vi "User Message Event Callback.vi"(4 "TS UI Data":T1, 5 "Event Data":cluster{"uiMsg":refnum<k7>}, 6 "Control Ref":refnum<k7>, 7 "Event Common Data":T2) -> ()   [LabVIEW 2015]
uses:
  Type defs/TS UI Data.ctl
  Type defs/Nest cluster.ctl
panel:
  # "SCANNED DATA"
  # "ITAC DATA"
  # "DoIP DATA"
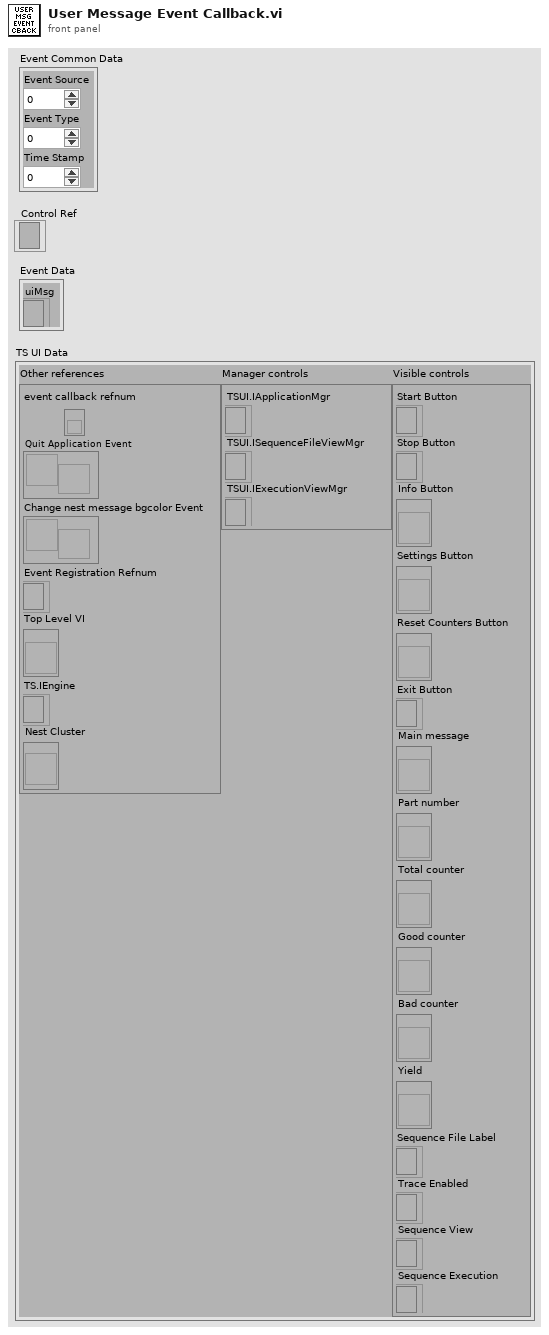
[diagram p1: front panel]
types:
  T1 = typedef "TS UI Data.ctl" = cluster{"Other references":cluster{"event callback refnum":refnum<k27>, "Quit Application Event":refnum<user-event>, "Change nest message bgcolor Event":refnum<user-event>, "event registration refnum":refnum<event-registration>, "Top Level VI":refnum<vi>, "TS.IEngine":refnum<k7>, "Nest Cluster":refnum<vi>}, "Manager controls":cluster{"TSUI.IApplicationMgr":refnum<k7>, "TSUI.ISequenceFileViewMgr":refnum<k7>, "TSUI.IExecutionViewMgr":refnum<k7>}, "Visible controls":cluster{"Start Button":refnum<k7>, "Stop Button":refnum<k7>, "Info Button":refnum<vi>, "Settings Button":refnum<vi>, "Reset Counters Button":refnum<vi>, "Exit Button":refnum<k7>, "Main message":refnum<vi>, "Part number":refnum<vi>, "Total counter":refnum<vi>, "Good counter":refnum<vi>, "Bad counter":refnum<vi>, "Yield":refnum<vi>, "Sequence File Label":refnum<k7>, "Trace Enabled":refnum<k7>, "Sequence View":refnum<k7>, "Sequence Execution":refnum<k7>}}
  T2 = cluster{"Event Source":i32, "Event Type":u32, "Time Stamp":u32}
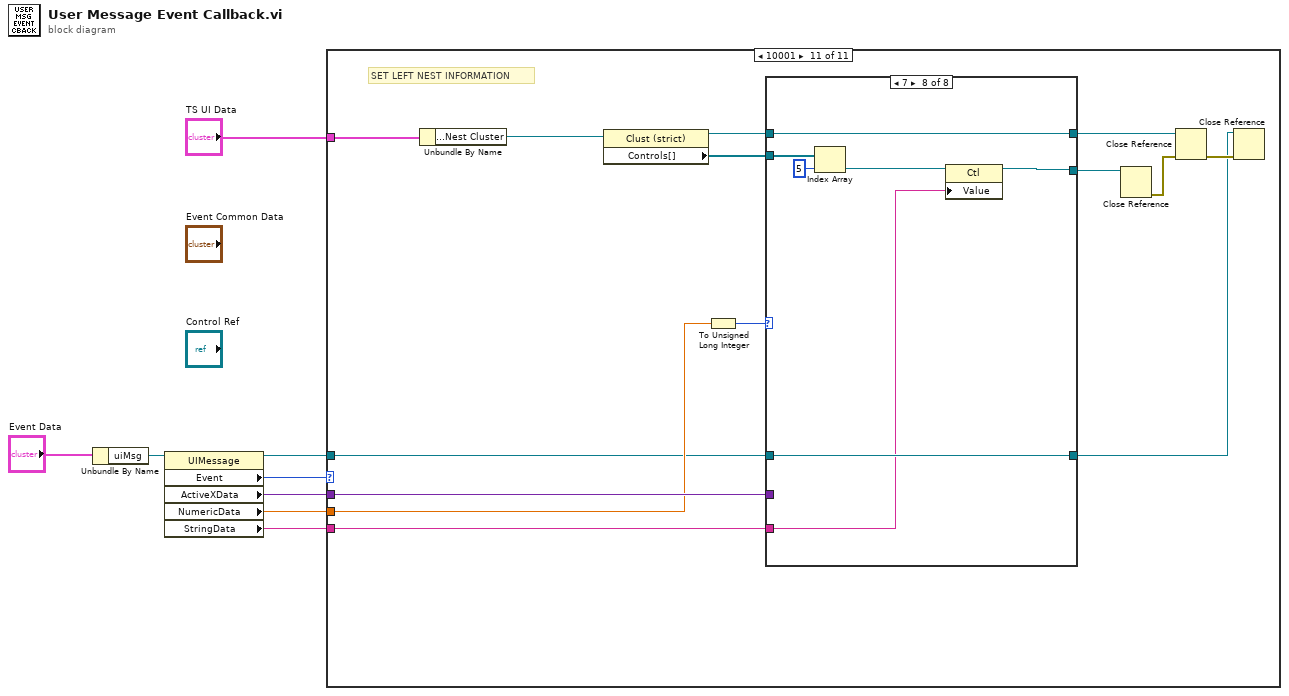
[diagram p0: block diagram]
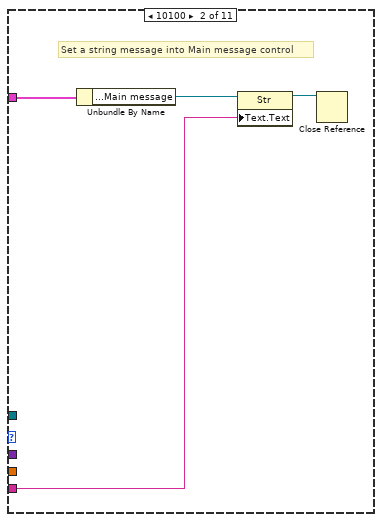
[diagram p3: hidden frame]
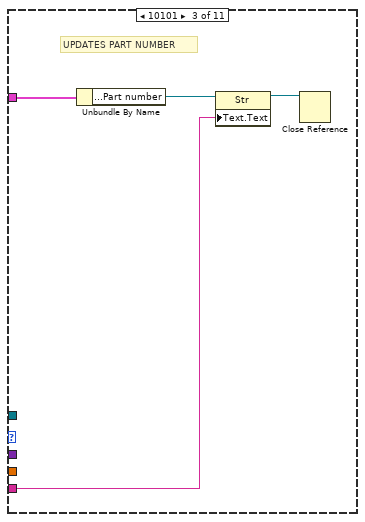
[diagram p4: hidden frame]
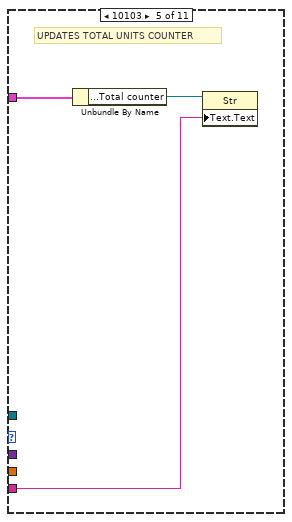
[diagram p6: hidden frame]
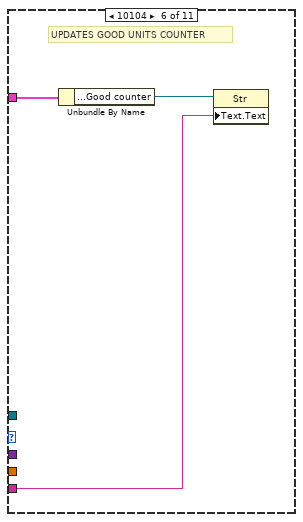
[diagram p7: hidden frame]
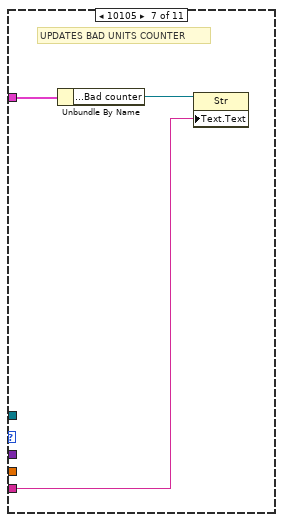
[diagram p8: hidden frame]
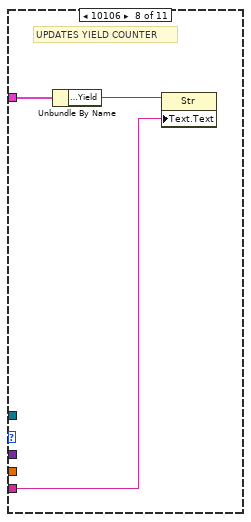
[diagram p9: hidden frame]
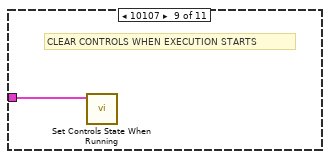
[diagram p10: hidden frame]
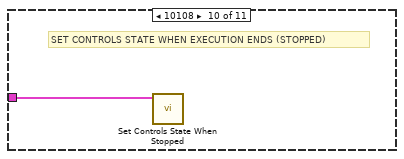
[diagram p11: hidden frame]
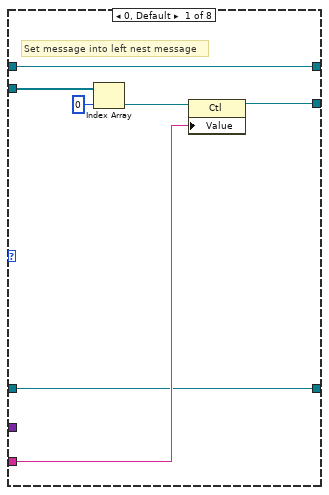
[diagram p12: hidden frame]
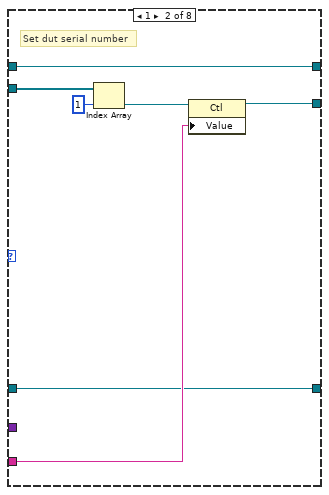
[diagram p13: hidden frame]
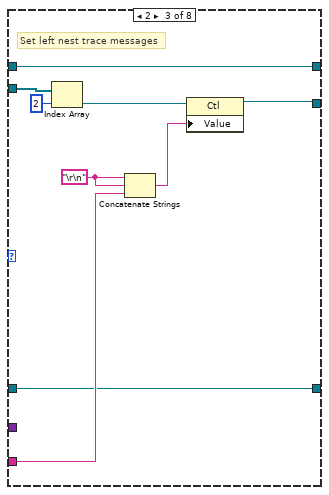
[diagram p14: hidden frame]
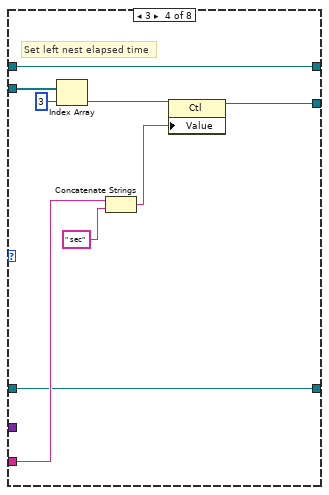
[diagram p15: hidden frame]
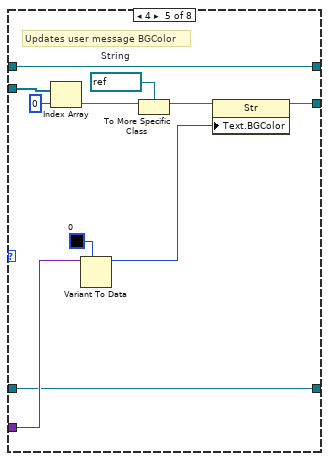
[diagram p16: hidden frame]
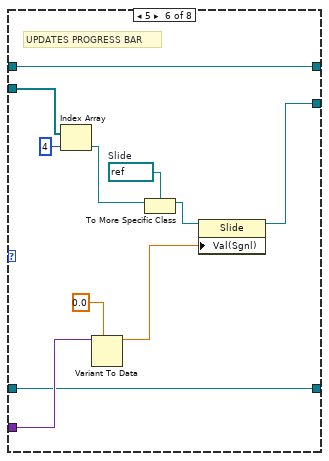
[diagram p17: hidden frame]
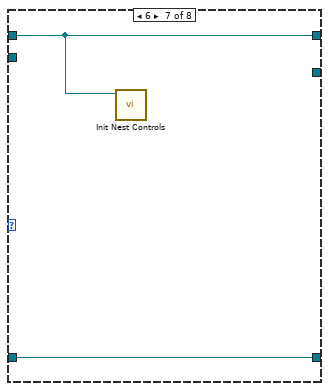
[diagram p18: hidden frame]
diagram:
  n1 = Unbundle By Name("Event Data") -> ("uiMsg"=w7:refnum<k7>)
  n2 = property class="UIMessage"(reference=w7) -> (reference out=w1:refnum<k7>, "Event"=w6:i32, "ActiveXData"=w3:variant, "NumericData"=w2:dbl, "StringData"=w4:string)  [unwired: 1 in, 1 out]
  n3 = case shown="10001" w6 {
    tunnel: "TS UI Data" -> [_ w12 w16 _ w19 w22 w25 w28 w29 w30 w44]
    tunnel: w4 -> [_ w9 w14 _ w17 w20 w23 w26 _ _ w38]
    tunnel: w3 -> [_ _ _ _ _ _ _ _ _ _ w43]
    tunnel: w2 -> [_ _ _ _ _ _ _ _ _ _ w42]
    tunnel: w1 -> [_ _ _ _ _ _ _ _ _ _ w34]
    frame 0, Default {
    }
    frame 10100 {
      # "Set a string message into Main message control"
      n4 = Unbundle By Name(w12) -> ("Visible controls.Main message"=w11:refnum<vi>)
      n5 = property class="Str"(reference=w11, "Text.Text"=w9) -> (reference out=w10:refnum<vi>)  [unwired: 1 in, 1 out]
      n6 = Close Reference(reference=w10) -> ()  [unwired: 1 in, 1 out]
    }
    frame 10101 {
      # "UPDATES PART NUMBER"
      n7 = Unbundle By Name(w16) -> ("Visible controls.Part number"=w15:refnum<vi>)
      n8 = property class="Str"(reference=w15, "Text.Text"=w14) -> (reference out=w13:refnum<vi>)  [unwired: 1 in, 1 out]
      n9 = Close Reference(reference=w13) -> ()  [unwired: 1 in, 1 out]
    }
    frame 10102 {
      # "UPDATES WORK ORDER"
    }
    frame 10103 {
      # "UPDATES TOTAL UNITS COUNTER"
      n10 = Unbundle By Name(w19) -> ("Visible controls.Total counter"=w18:refnum<vi>)
      n11 = property class="Str"(reference=w18, "Text.Text"=w17) -> ()  [unwired: 1 in, 2 out]
    }
    frame 10104 {
      # "UPDATES GOOD UNITS COUNTER"
      n12 = Unbundle By Name(w22) -> ("Visible controls.Good counter"=w21:refnum<vi>)
      n13 = property class="Str"(reference=w21, "Text.Text"=w20) -> ()  [unwired: 1 in, 2 out]
    }
    frame 10105 {
      # "UPDATES BAD UNITS COUNTER"
      n14 = Unbundle By Name(w25) -> ("Visible controls.Bad counter"=w24:refnum<vi>)
      n15 = property class="Str"(reference=w24, "Text.Text"=w23) -> ()  [unwired: 1 in, 2 out]
    }
    frame 10106 {
      # "UPDATES YIELD COUNTER"
      n16 = Unbundle By Name(w28) -> ("Visible controls.Yield"=w27:refnum<vi>)
      n17 = property class="Str"(reference=w27, "Text.Text"=w26) -> ()  [unwired: 1 in, 2 out]
    }
    frame 10107 {
      # "CLEAR CONTROLS WHEN EXECUTION STARTS"
      n18 = call "Set Controls State When Running.vi"("TS UI Data in"=w29) -> ()  [unwired: 10 in, 1 out]
    }
    frame 10108 {
      # "SET CONTROLS STATE WHEN EXECUTION ENDS (STOPPED)"
      n19 = call "Set Controls State When Stopped.vi"("TS UI Data in"=w30) -> ()  [unwired: 10 in, 1 out]
    }
    frame 10001 {
      # "SET LEFT NEST INFORMATION"
      n20 = Unbundle By Name(w44) -> ("Other references.Nest Cluster"=w40:refnum<vi>)
      n21 = property class="Clust (strict)"(reference=w40) -> (reference out=w32:refnum<vi>, "Controls[]"=w39:refnum<vi>[])  [unwired: 1 in, 1 out]
      n22 = To Unsigned Long Integer(number=w42) -> (unsigned 32bit integer=w41:u32)
      n23 = case shown="7" w41 {
        tunnel: w43 -> [_ _ _ _ w86 w96 _ _]
        tunnel: w39 -> [w49 w56 w67 w76 w83 w97 _ w107]
        tunnel: w38 -> [w48 w55 w63 w72 _ _ _ w101]
        tunnel: [w45 w52 w59 w68 w77 w91 _ w104] -> w35
        tunnel: w34 -> [w46 w53 w60 w70 w84 w93 w100 w103]
        tunnel: [w46 w53 w60 w70 w84 w93 w100 w103] -> w33
        tunnel: w32 -> [w47 w54 w61 w69 w85 w92 w99 w102]
        tunnel: [w47 w54 w61 w69 w85 w92 w99 w102] -> w31
        frame 0, Default {
          # "Set message into left nest message"
          n24 = Index Array(array=w49, index=0) -> (element=w50:refnum<vi>)
          n25 = property class="Ctl"(reference=w50, "Value"=w48) -> (reference out=w45:refnum<vi>)  [unwired: 1 in, 1 out]
        }
        frame 1 {
          # "Set dut serial number"
          n26 = Index Array(array=w56, index=1) -> (element=w57:refnum<vi>)
          n27 = property class="Ctl"(reference=w57, "Value"=w55) -> (reference out=w52:refnum<vi>)  [unwired: 1 in, 1 out]
        }
        frame 2 {
          w62 = "\r\n"
          # "Set left nest trace messages"
          n28 = Index Array(array=w67, index=2) -> (element=w65:refnum<vi>)
          n29 = Concatenate Strings(w62, w62, w63) -> (w64:string)
          n30 = property class="Ctl"(reference=w65, "Value"=w64) -> (reference out=w59:refnum<vi>)  [unwired: 1 in, 1 out]
        }
        frame 3 {
          # "Set left nest elapsed time"
          n31 = Index Array(array=w76, index=3) -> (element=w74:refnum<vi>)
          n32 = Concatenate Strings(w72, " sec" ("string")) -> (w73:string)
          n33 = property class="Ctl"(reference=w74, "Value"=w73) -> (reference out=w68:refnum<vi>)  [unwired: 1 in, 1 out]
        }
        frame 4 {
          w80 = refnum<vi> refnum  # String
          # "Updates user message BGColor"
          n34 = Index Array(array=w83, index=0) -> (element=w81:refnum<vi>)
          n35 = Variant To Data(type=u32 0, Variant=w86) -> (data=w78:u32)  [unwired: 1 in, 1 out]
          n36 = To More Specific Class(target class=w80, reference=w81) -> (specific class reference=w79:refnum<vi>)  [unwired: 1 in, 1 out]
          n37 = property class="Str"(reference=w79, "Text.BGColor"=w78) -> (reference out=w77:refnum<vi>)  [unwired: 1 in, 1 out]
        }
        frame 5 {
          w90 = refnum<vi> refnum  # Slide
          # "UPDATES PROGRESS BAR"
          n38 = Index Array(array=w97, index=4) -> (element=w89:refnum<vi>)
          n39 = Variant To Data(type=0.0, Variant=w96) -> (data=w94:dbl)  [unwired: 1 in, 1 out]
          n40 = To More Specific Class(target class=w90, reference=w89) -> (specific class reference=w88:refnum<vi>)  [unwired: 1 in, 1 out]
          n41 = property class="Slide"(reference=w88, "Val(Sgnl)"=w94) -> (reference out=w91:refnum<vi>)  [unwired: 1 in, 1 out]
        }
        frame 6 {
          n42 = call "Init Nest Controls.vi"("Nest Cluster"=w99) -> ()  [unwired: 10 in, 1 out]
        }
        frame 7 {
          n43 = Index Array(array=w107, index=5) -> (element=w105:refnum<vi>)
          n44 = property class="Ctl"(reference=w105, "Value"=w101) -> (reference out=w104:refnum<vi>)  [unwired: 1 in, 1 out]
        }
      }
      n45 = Close Reference(reference=w35) -> (error out=w37:errorcluster)  [unwired: 1 in]
      n46 = Close Reference(reference=w31, error in (no error)=w37) -> (error out=w36:errorcluster)
      n47 = Close Reference(reference=w33, error in (no error)=w36) -> ()  [unwired: 1 out]
    }
  }
